vi "ClassAppData.Load INI File.vi"(8 "error in (no error)":errorcluster, 9 "Sections that List RemoteFile":string[](array[string]), 10 "INI File":path, 11 "Class - App Data in":refnum<class "Class.AppData.lvclass">) -> (0 "error out":errorcluster, 2 "Additional Cfg Files":path[](array[path]), 3 "Class - App Data out":refnum<class "Class.AppData.lvclass">)   [LabVIEW 2024, in "EQMF.lvlib" / "Config Utils.lvlib" / "Class.AppData.lvclass"]
doc: "<B>AppData Class:</B>\nThe AppData class keeps track of a library of data items that are used by an application. These data items have a name (text string) and value that can be any data type. \n\n<B>AppData.Load INI VI:</B>\nThis VI reads INI files and stores the items in the INI files to the data library. All data types read form the INI file are treated as strings. The names of the items read are the section name concatenated wit the item name separated by a period.\n\n<B>EXAMPLE:</B>\nINI File contents is\n[SectionX]\nItemY = \"AABBCC\"\nItemZ = 1234\n\nThe items in the data library will be\nSectionX.ItemY = \"AABBCC\"\nSectionX.ItemZ = \"1234\"\n\nThe input <B>Sections that List RemoteFile</B> is an array of string. This is a list of INI file sections that contain a list of additional config files to be read. Any items in those sections will be treated as paths to additional INI files and those files will be read, and their contents added to the Data Library. Those INI files may also have sections that point to additional files to be read."
uses:
  Class.AppData.lvclass
  Class.AppData.lvclass/Class.AppData.ctl
panel:
  in  "Init (Remove Previous Data)":bool
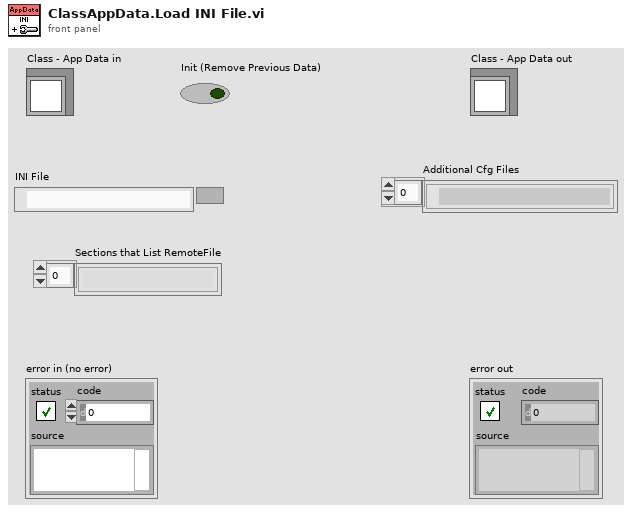
[diagram p1: front panel]
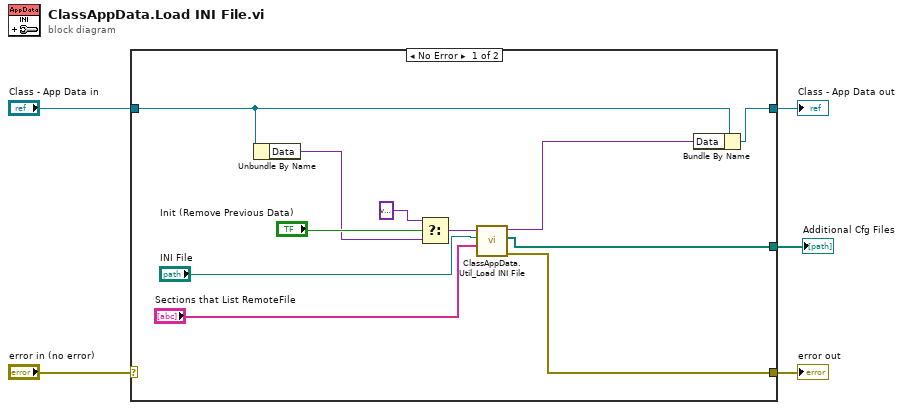
[diagram p0: block diagram]
diagram:
  n1 = case shown="No Error" "error in (no error)" {
    selector: "error in (no error)" -> [_ w18]
    tunnel: [w14 w18] -> w4
    tunnel: [w16 w17] -> w2
    tunnel: "Class - App Data in" -> [w15 w17]
    tunnel: [w6 _] -> w1
    frame No Error {
      n2 = Unbundle By Name(w15) -> ("Data"=w11:variant)
      n3 = Select(t=variant, s="Init (Remove Previous Data)", f=w11) -> (s? t:f=w8:variant)
      n4 = call "ClassAppData.Util_Load INI File.vi"("RmtFileSect"="Sections that List RemoteFile", "Input INI"="INI File", "Data In"=w8) -> ("error out"=w14:errorcluster, "Additional Cfg Files"=w6:path[], "Data Out"=w13:variant)  [unwired: 6 in]
      n5 = Bundle By Name(cluster=w15, "Data"=w13) -> (w16:refnum<class "Class.AppData.lvclass">)
    }
    frame Error {
    }
  }
  "error out" <- w4
  "Class - App Data out" <- w2
  "Additional Cfg Files" <- w1
